vi "Get_Set_Status_Errors.vi"(8 "Status/Errors in":refnum<vi>, 9 "Value in":variant, 10 "Element":T1=enum."Errors", 11 "Set?":bool) -> (0 "Status/Errors out":refnum<vi>, 1 "Value out":variant)   [LabVIEW 2010]
uses:
  Controls/Status_Errors_Elements.ctl
  Controls/TabPage_Errors.ctl
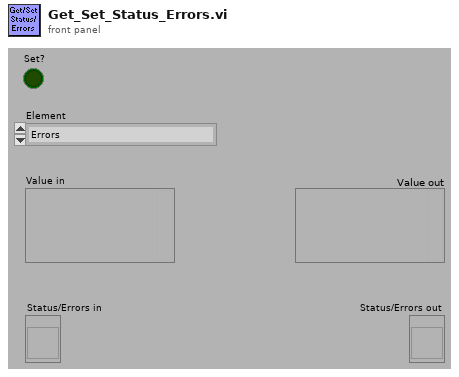
[diagram p1: front panel]
types:
  T1 = typedef "Status_Errors_Elements.ctl" = enum16{"Default", "Errors", "Master status", "Slave status", "Master connected?", "Slave connected?", "Master GPS on board?", "Slave GPS on board?", "Master: slave detected?", "Slave: slave detected?", "Last message from master", "Last message from slave", "Master temperature"}
  T2 = typedef "Semaphore RefNum" = refnum<k1>
  T3 = typedef "TabPage_Errors.ctl" = cluster{"Errors":string, "Connected?_MAS":bool, "Status_Errors_MAS":bool, "GPS?_MAS":bool, "Slave?_MAS":bool, "Last_Message_MAS":timestamp, "Temperature_MAS":sgl, "Connected?_SLV":bool, "Status_Errors_SLV":bool, "GPS?_SLV":bool, "Slave?_SLV":bool, "Last_Message_SLV":timestamp}
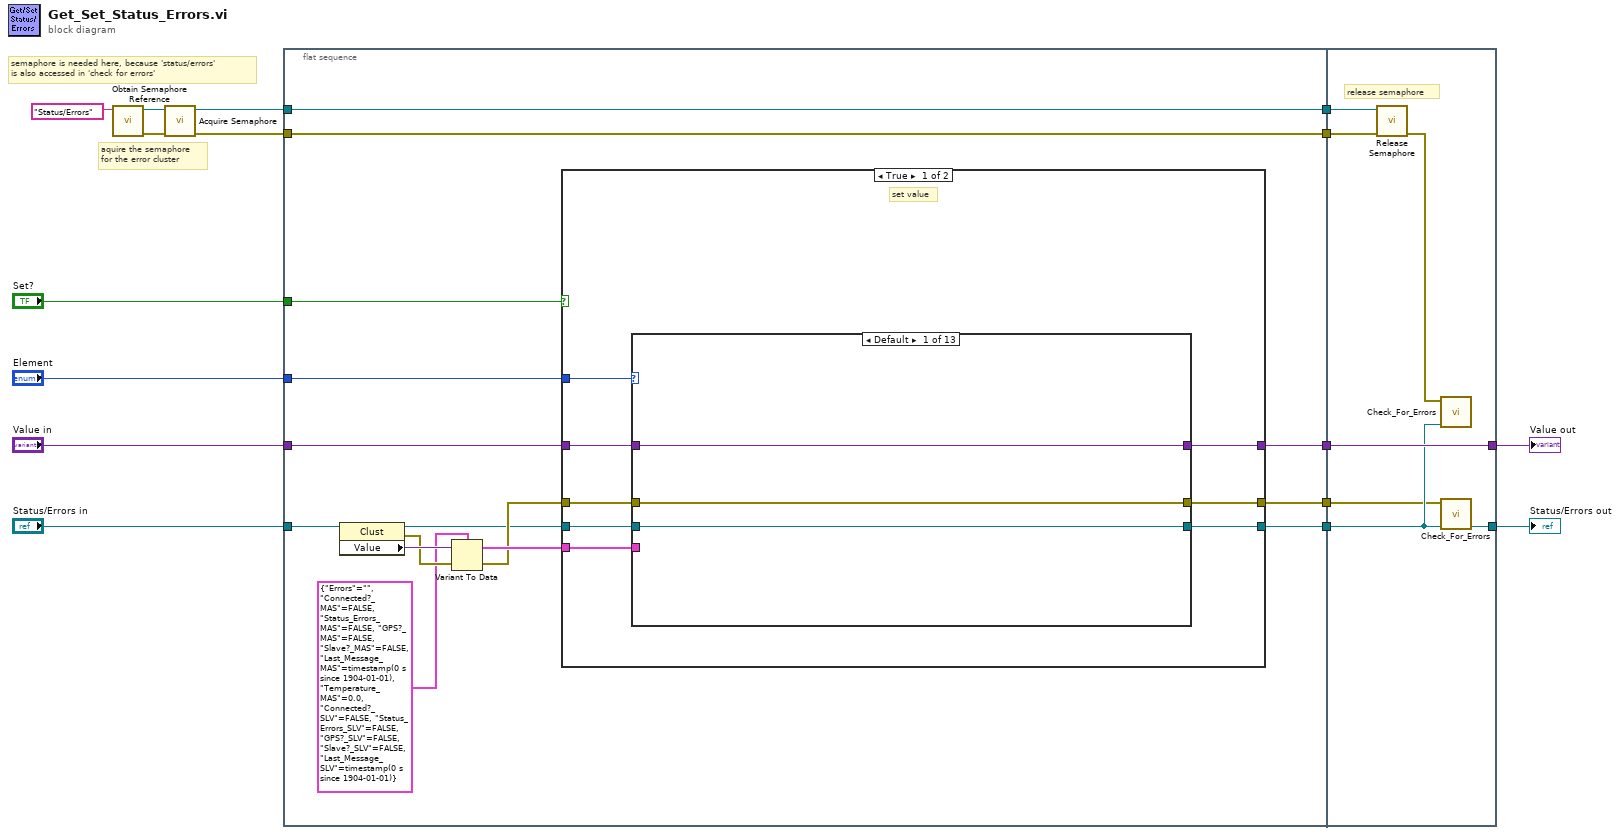
[diagram p0: block diagram]
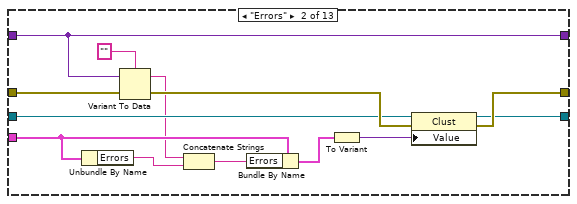
[diagram p2: hidden frame]
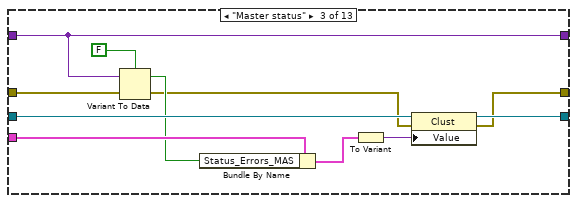
[diagram p3: hidden frame]
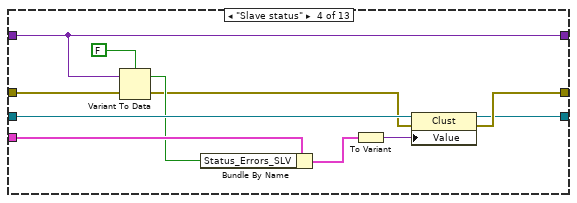
[diagram p4: hidden frame]
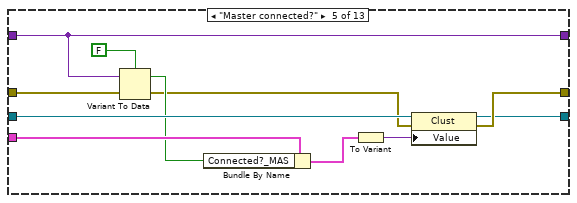
[diagram p5: hidden frame]
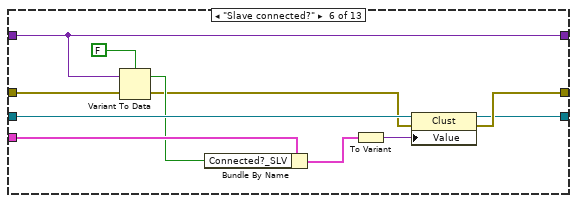
[diagram p6: hidden frame]
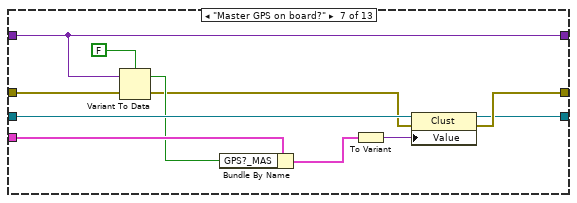
[diagram p7: hidden frame]
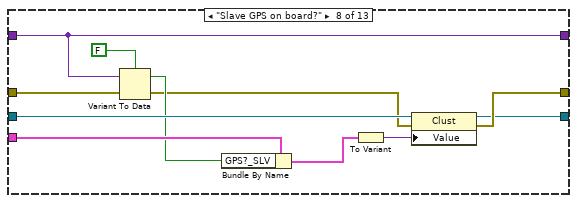
[diagram p8: hidden frame]
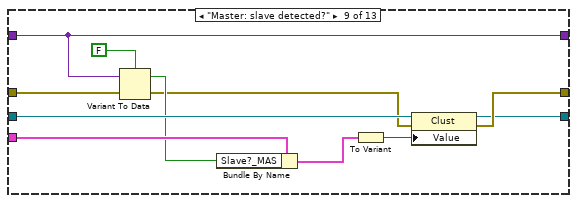
[diagram p9: hidden frame]
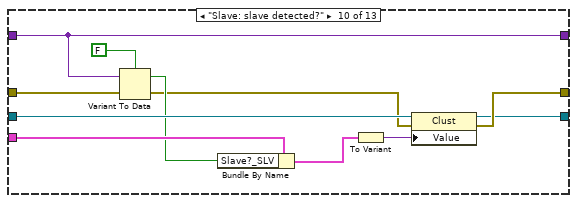
[diagram p10: hidden frame]
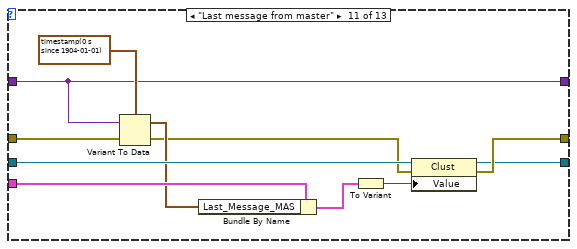
[diagram p11: hidden frame]
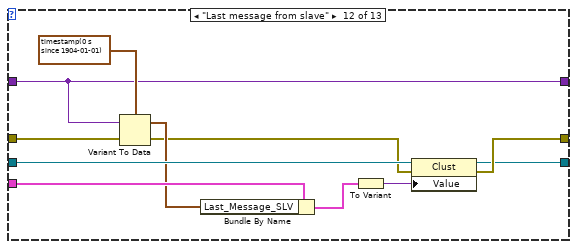
[diagram p12: hidden frame]
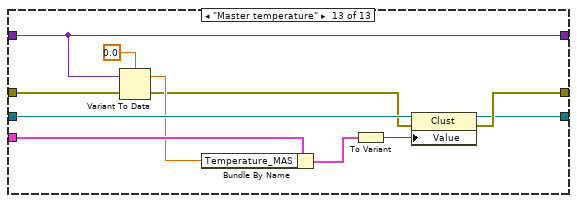
[diagram p13: hidden frame]
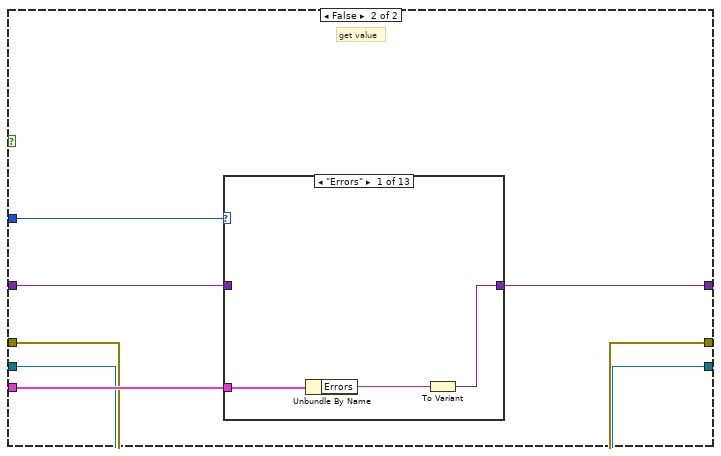
[diagram p14: hidden frame]
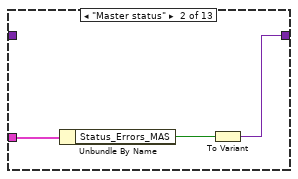
[diagram p15: hidden frame]
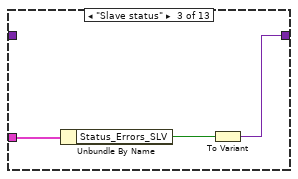
[diagram p16: hidden frame]
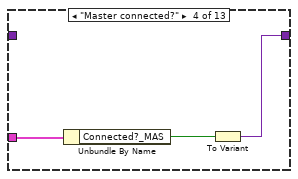
[diagram p17: hidden frame]
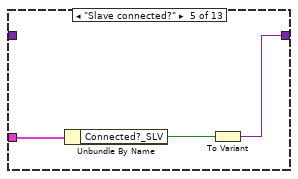
[diagram p18: hidden frame]
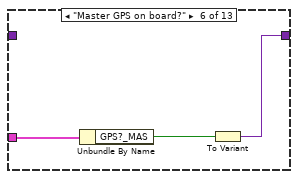
[diagram p19: hidden frame]
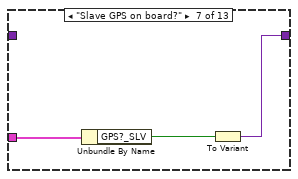
[diagram p20: hidden frame]
diagram:
  # "semaphore is needed here, because 'status/errors'\nis also accessed in 'check for errors'"
  # "aquire the semaphore\nfor the error cluster"
  n1 = call <vilib>:"Obtain Semaphore Reference.vi"("name (unnamed)"="Status/Errors") -> ("error out"=w11:errorcluster, "semaphore"=w10:T2)  [unwired: 2 in, 3 out]
  n2 = call <vilib>:"Acquire Semaphore.vi"("error in (no error)"=w11, "semaphore"=w10) -> ("error out"=w5:errorcluster, "semaphore out"=w3:T2)  [unwired: 1 in, 3 out]
  n3 = flat-sequence {
    tunnel: "Element" -> [w28]
    tunnel: "Value in" -> [w26]
    tunnel: "Set?" -> [w23]
    tunnel: "Status/Errors in" -> [w21]
    tunnel: [w22] -> w7
    tunnel: [w20] -> w6
    tunnel: w5 -> [w20]
    tunnel: [w19] -> w4
    tunnel: w3 -> [w19]
    tunnel: [w18] -> w2
    tunnel: [w17] -> w1
    tunnel: [w226] -> w12
    tunnel: [w225] -> w14
    tunnel: w7 -> [w226]
    tunnel: w6 -> [w224]
    tunnel: w4 -> [w223]
    tunnel: w2 -> [w221]
    tunnel: w1 -> [w220]
    frame #0 {
      n4 = property class="Clust"(reference=w21) -> (reference out=w24:refnum<vi>, error out=w30:errorcluster, "Value"=w31:variant)  [unwired: 1 in]
      n5 = Variant To Data(error in=w30, Variant=w31, type=T3 {"Errors"="", "Connected?_MAS"=FALSE, "Status_Errors_MAS"=FALSE, "GPS?_MAS"=FALSE, "Slave?_MAS"=FALSE, "Last_Message_MAS"=timestamp(0 s since 1904-01-01), "Temperature_MAS"=0.0, "Connected?_SLV"=FALSE, "Status_Errors_SLV"=FALSE, "GPS?_SLV"=FALSE, "Slave?_SLV"=FALSE, "Last_Message_SLV"=timestamp(0 s since 1904-01-01)} ("GEN_Page_Statistics")) -> (error out=w25:errorcluster, data=w27:T3)
      n6 = case shown="True" w23 {
        tunnel: w28 -> [w39 w182]
        tunnel: w27 -> [w38 w181]
        tunnel: w26 -> [w37 w177]
        tunnel: w25 -> [w36 w180]
        tunnel: w24 -> [w35 w178]
        tunnel: [w34 w178] -> w18
        tunnel: [w33 w180] -> w17
        tunnel: [w32 w179] -> w22
        frame True {
          # "set value"
          n7 = case shown="Default" w39 {
            tunnel: w38 -> [_ w50 w66 w77 w88 w99 w110 w121 w132 w143 w154 w165 w176]
            tunnel: w37 -> [w40 w47 w56 w67 w78 w89 w100 w111 w122 w133 w144 w155 w166]
            tunnel: w36 -> [w41 w55 w65 w76 w87 w98 w109 w120 w131 w142 w153 w164 w175]
            tunnel: w35 -> [w42 w45 w64 w75 w86 w97 w108 w119 w130 w141 w152 w163 w174]
            tunnel: [w42 w46 w60 w68 w79 w90 w101 w112 w123 w134 w145 w156 w167] -> w34
            tunnel: [w41 w51 w57 w69 w80 w91 w102 w113 w124 w135 w146 w157 w168] -> w33
            tunnel: [w40 w47 w56 w67 w78 w89 w100 w111 w122 w133 w144 w155 w166] -> w32
            frame Default {
            }
            frame "Errors" {
              n8 = Unbundle By Name(w50) -> ("Errors"=w49:string)
              n9 = Variant To Data(error in=w55, Variant=w47, type="") -> (error out=w53:errorcluster, data=w44:string)
              n10 = Concatenate Strings(w44, w49) -> (w43:string)
              n11 = Bundle By Name(cluster=w50, "Errors"=w43) -> (w54:T3)
              n12 = To Variant(anything=w54) -> (Variant=w48:variant)
              n13 = property class="Clust"(reference=w45, error in=w53, "Value"=w48) -> (reference out=w46:refnum<vi>, error out=w51:errorcluster)
            }
            frame "Master status" {
              n14 = Variant To Data(error in=w65, Variant=w56, type=FALSE) -> (error out=w58:errorcluster, data=w62:bool)
              n15 = Bundle By Name(cluster=w66, "Status_Errors_MAS"=w62) -> (w63:T3)
              n16 = To Variant(anything=w63) -> (Variant=w59:variant)
              n17 = property class="Clust"(reference=w64, error in=w58, "Value"=w59) -> (reference out=w60:refnum<vi>, error out=w57:errorcluster)
            }
            frame "Slave status" {
              n18 = Variant To Data(error in=w76, Variant=w67, type=FALSE) -> (error out=w71:errorcluster, data=w72:bool)
              n19 = Bundle By Name(cluster=w77, "Status_Errors_SLV"=w72) -> (w74:T3)
              n20 = To Variant(anything=w74) -> (Variant=w73:variant)
              n21 = property class="Clust"(reference=w75, error in=w71, "Value"=w73) -> (reference out=w68:refnum<vi>, error out=w69:errorcluster)
            }
            frame "Master connected?" {
              n22 = Variant To Data(error in=w87, Variant=w78, type=FALSE) -> (error out=w82:errorcluster, data=w83:bool)
              n23 = Bundle By Name(cluster=w88, "Connected?_MAS"=w83) -> (w85:T3)
              n24 = To Variant(anything=w85) -> (Variant=w84:variant)
              n25 = property class="Clust"(reference=w86, error in=w82, "Value"=w84) -> (reference out=w79:refnum<vi>, error out=w80:errorcluster)
            }
            frame "Slave connected?" {
              n26 = Variant To Data(error in=w98, Variant=w89, type=FALSE) -> (error out=w93:errorcluster, data=w94:bool)
              n27 = Bundle By Name(cluster=w99, "Connected?_SLV"=w94) -> (w96:T3)
              n28 = To Variant(anything=w96) -> (Variant=w95:variant)
              n29 = property class="Clust"(reference=w97, error in=w93, "Value"=w95) -> (reference out=w90:refnum<vi>, error out=w91:errorcluster)
            }
            frame "Master GPS on board?" {
              n30 = Variant To Data(error in=w109, Variant=w100, type=FALSE) -> (error out=w104:errorcluster, data=w105:bool)
              n31 = Bundle By Name(cluster=w110, "GPS?_MAS"=w105) -> (w107:T3)
              n32 = To Variant(anything=w107) -> (Variant=w106:variant)
              n33 = property class="Clust"(reference=w108, error in=w104, "Value"=w106) -> (reference out=w101:refnum<vi>, error out=w102:errorcluster)
            }
            frame "Slave GPS on board?" {
              n34 = Variant To Data(error in=w120, Variant=w111, type=FALSE) -> (error out=w115:errorcluster, data=w116:bool)
              n35 = Bundle By Name(cluster=w121, "GPS?_SLV"=w116) -> (w118:T3)
              n36 = To Variant(anything=w118) -> (Variant=w117:variant)
              n37 = property class="Clust"(reference=w119, error in=w115, "Value"=w117) -> (reference out=w112:refnum<vi>, error out=w113:errorcluster)
            }
            frame "Master: slave detected?" {
              n38 = Variant To Data(error in=w131, Variant=w122, type=FALSE) -> (error out=w126:errorcluster, data=w127:bool)
              n39 = Bundle By Name(cluster=w132, "Slave?_MAS"=w127) -> (w129:T3)
              n40 = To Variant(anything=w129) -> (Variant=w128:variant)
              n41 = property class="Clust"(reference=w130, error in=w126, "Value"=w128) -> (reference out=w123:refnum<vi>, error out=w124:errorcluster)
            }
            frame "Slave: slave detected?" {
              n42 = Variant To Data(error in=w142, Variant=w133, type=FALSE) -> (error out=w137:errorcluster, data=w138:bool)
              n43 = Bundle By Name(cluster=w143, "Slave?_SLV"=w138) -> (w140:T3)
              n44 = To Variant(anything=w140) -> (Variant=w139:variant)
              n45 = property class="Clust"(reference=w141, error in=w137, "Value"=w139) -> (reference out=w134:refnum<vi>, error out=w135:errorcluster)
            }
            frame "Last message from master" {
              n46 = Variant To Data(error in=w153, Variant=w144, type=timestamp(0 s since 1904-01-01) ("Last message from master")) -> (error out=w147:errorcluster, data=w148:timestamp)
              n47 = Bundle By Name(cluster=w154, "Last_Message_MAS"=w148) -> (w151:T3)
              n48 = To Variant(anything=w151) -> (Variant=w150:variant)
              n49 = property class="Clust"(reference=w152, error in=w147, "Value"=w150) -> (reference out=w145:refnum<vi>, error out=w146:errorcluster)
            }
            frame "Last message from slave" {
              n50 = Variant To Data(error in=w164, Variant=w155, type=timestamp(0 s since 1904-01-01) ("Last message from master")) -> (error out=w158:errorcluster, data=w159:timestamp)
              n51 = Bundle By Name(cluster=w165, "Last_Message_SLV"=w159) -> (w162:T3)
              n52 = To Variant(anything=w162) -> (Variant=w161:variant)
              n53 = property class="Clust"(reference=w163, error in=w158, "Value"=w161) -> (reference out=w156:refnum<vi>, error out=w157:errorcluster)
            }
            frame "Master temperature" {
              n54 = Variant To Data(error in=w175, Variant=w166, type=sgl 0.0 ("Last message from master")) -> (error out=w169:errorcluster, data=w170:sgl)
              n55 = Bundle By Name(cluster=w176, "Temperature_MAS"=w170) -> (w173:T3)
              n56 = To Variant(anything=w173) -> (Variant=w172:variant)
              n57 = property class="Clust"(reference=w174, error in=w169, "Value"=w172) -> (reference out=w167:refnum<vi>, error out=w168:errorcluster)
            }
          }
        }
        frame False {
          # "get value"
          n58 = case shown="\"Errors\"" w182 {
            tunnel: w181 -> [w185 w188 w191 w194 w197 w200 w203 w206 w209 w212 w215 w218 _]
            tunnel: [w183 w186 w189 w192 w195 w198 w201 w204 w207 w210 w213 w216 w219] -> w179
            tunnel: w177 -> [_ _ _ _ _ _ _ _ _ _ _ _ w219]
            frame "Errors" {
              n59 = Unbundle By Name(w185) -> ("Errors"=w184:string)
              n60 = To Variant(anything=w184) -> (Variant=w183:variant)
            }
            frame "Master status" {
              n61 = Unbundle By Name(w188) -> ("Status_Errors_MAS"=w187:bool)
              n62 = To Variant(anything=w187) -> (Variant=w186:variant)
            }
            frame "Slave status" {
              n63 = Unbundle By Name(w191) -> ("Status_Errors_SLV"=w190:bool)
              n64 = To Variant(anything=w190) -> (Variant=w189:variant)
            }
            frame "Master connected?" {
              n65 = Unbundle By Name(w194) -> ("Connected?_MAS"=w193:bool)
              n66 = To Variant(anything=w193) -> (Variant=w192:variant)
            }
            frame "Slave connected?" {
              n67 = Unbundle By Name(w197) -> ("Connected?_SLV"=w196:bool)
              n68 = To Variant(anything=w196) -> (Variant=w195:variant)
            }
            frame "Master GPS on board?" {
              n69 = Unbundle By Name(w200) -> ("GPS?_MAS"=w199:bool)
              n70 = To Variant(anything=w199) -> (Variant=w198:variant)
            }
            frame "Slave GPS on board?" {
              n71 = Unbundle By Name(w203) -> ("GPS?_SLV"=w202:bool)
              n72 = To Variant(anything=w202) -> (Variant=w201:variant)
            }
            frame "Master: slave detected?" {
              n73 = Unbundle By Name(w206) -> ("Slave?_MAS"=w205:bool)
              n74 = To Variant(anything=w205) -> (Variant=w204:variant)
            }
            frame "Slave: slave detected?" {
              n75 = Unbundle By Name(w209) -> ("Slave?_SLV"=w208:bool)
              n76 = To Variant(anything=w208) -> (Variant=w207:variant)
            }
            frame "Last message from master" {
              n77 = Unbundle By Name(w212) -> ("Last_Message_MAS"=w211:timestamp)
              n78 = To Variant(anything=w211) -> (Variant=w210:variant)
            }
            frame "Last message from slave" {
              n79 = Unbundle By Name(w215) -> ("Last_Message_SLV"=w214:timestamp)
              n80 = To Variant(anything=w214) -> (Variant=w213:variant)
            }
            frame "Master temperature" {
              n81 = Unbundle By Name(w218) -> ("Temperature_MAS"=w217:sgl)
              n82 = To Variant(anything=w217) -> (Variant=w216:variant)
            }
            frame Default {
            }
          }
        }
      }
    }
    frame #1 {
      # "release semaphore"
      n83 = call <vilib>:"Release Semaphore.vi"("error in (no error)"=w224, "semaphore"=w223) -> ("error out"=w222:errorcluster)  [unwired: 5 out]
      n84 = call "Check_For_Errors.vi"("Status/Errors in"=w221, "error in"=w222) -> ()  [unwired: 10 out]
      n85 = call "Check_For_Errors.vi"("Status/Errors in"=w221, "error in"=w220) -> ("Status/Errors out"=w225:refnum<vi>)  [unwired: 9 out]
    }
  }
  "Status/Errors out" <- w14
  "Value out" <- w12
